vi "Subpanel UI.vi"(8 "error in (no error)":errorcluster, 10 "Message Queue":refnum<queue>, 11 "Pump Controller in":refnum<class "Pump Controller.lvclass">) -> (0 "error out":errorcluster, 3 "Pump Controller out":refnum<class "Pump Controller.lvclass">)   [LabVIEW 2020, in "Pump Controller.lvclass"]
doc: "The UI that will be inserted into subpanels so data can be displayed to the user. The class will use an internally managed message queue to communicate to it. The user should only communicate to this UI through class methods."
uses:
  Pump Controller.lvclass
  Pump Controller.lvclass/Pump Controller.ctl
  Sub VIs/Message Queue/test Message Queue.lvlib
  Sub VIs/Message Queue/Enqueue Message (Single).vi
  <vilib>/Utility/error.llb/Error Cluster From Error Code.vi
  <vilib>/ErrorRing/Error Ring.xnode
  Sub VIs/Message Queue/Message Cluster.ctl
panel:
  out "Name":string
  out "Fault":bool
  out "Running?":bool
  out "Pressure (psi)":dbl format="%#.0f"
  out "Flow Rate (mL/min)":dbl format="%.3f"
  in  "Time Interval (sec)":i32=1200
  out "Pressure Graph":cluster{timestamp[], dbl[]}[](graph)
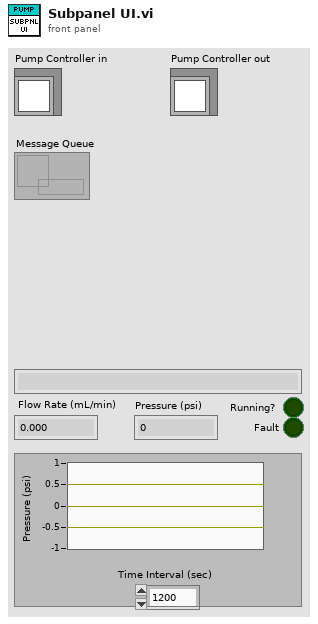
[diagram p1: front panel]
types:
  T1 = cluster{"Data Timestamps":timestamp[], "Data Values":dbl[], "Previous Run State":bool}
  T2 = typedef "Pump Controller.lvclass/Pump Controller State.ctl" = cluster{"VISA Resource":refnum<visa-resource-name>, "Flow Rate":dbl, "Running":bool, "Running Since":timestamp, "Pressure Data Point":cluster{"Time Stamp":timestamp, "Value":dbl}, "Fault":bool, "Sampling Rate (sec/sample)":dbl}
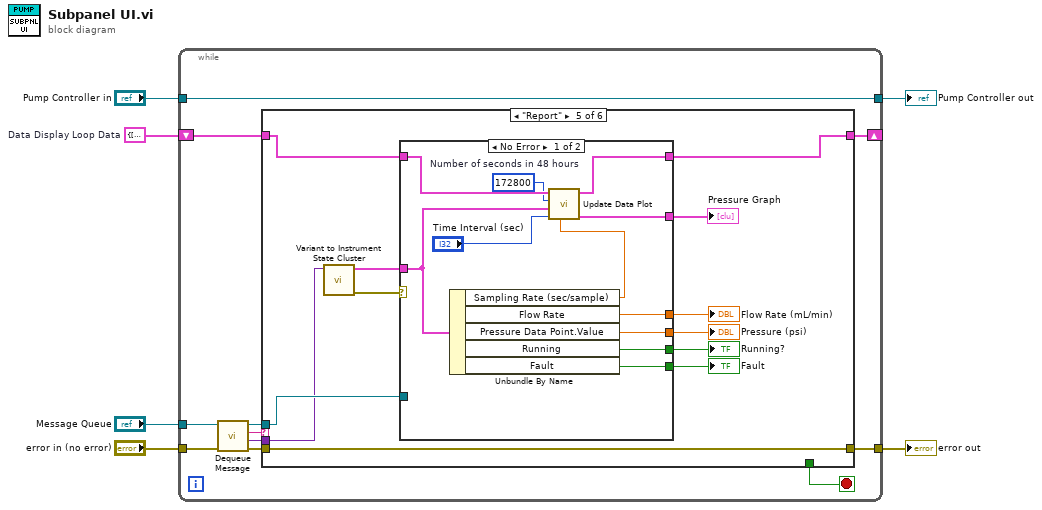
[diagram p0: block diagram]
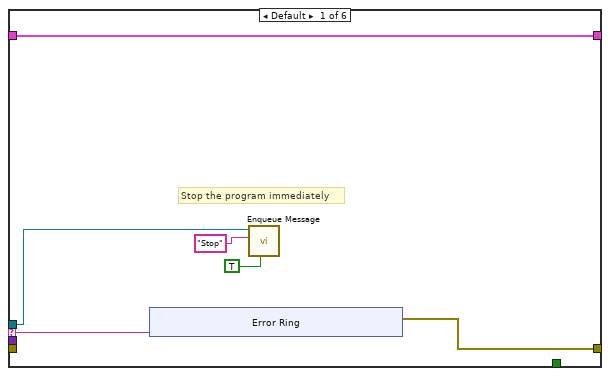
[diagram p2: hidden frame]
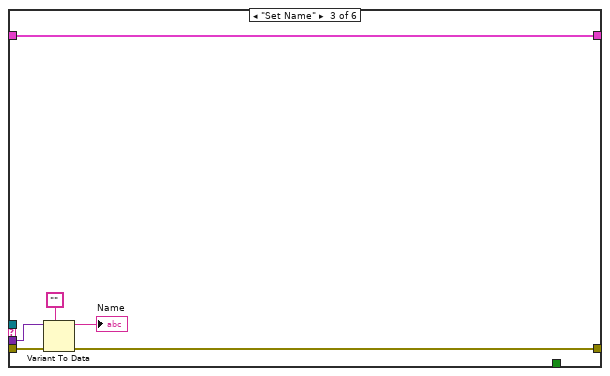
[diagram p4: hidden frame]
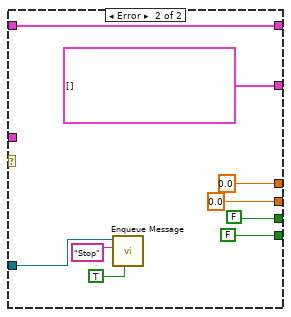
[diagram p6: hidden frame]
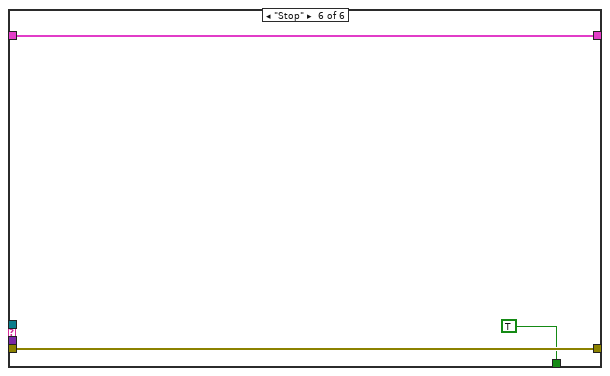
[diagram p7: hidden frame]
diagram:
  w1 = T1 {"Data Timestamps"=[], "Data Values"=[], "Previous Run State"=FALSE}  # Data Display Loop Data
  n1 = while {
    tunnel: [w7] -> w5
    tunnel: "Pump Controller in" -> [w7]
    tunnel: [w11] -> w3
    tunnel: "error in (no error)" -> [w17]
    tunnel: "Message Queue" -> [w16]
    shift-right: [w8] -> _
    shift-left: w1 -> [w9]
    stop <- w10 stop-if-true
    n2 = call "Dequeue Message.vi"("error in (no error)"=w17, "Message Queue"=w16) -> ("error out"=w12:errorcluster, "Message Data"=w14:variant, "Message"=w15:string, "dup Message Queue"=w13:refnum<queue>)  [unwired: 6 in]
    n3 = case shown="\"Report\"" w15 {
      selector: w15 -> [w19 _ _ _ _ _]
      tunnel: w14 -> [_ _ w35 _ w45 _]
      tunnel: w13 -> [w20 _ _ _ w47 _]
      tunnel: w12 -> [_ w32 w38 w40 w52 w75]
      tunnel: [w18 w32 w36 w40 w52 w75] -> w11
      tunnel: [_ _ _ _ _ TRUE] -> w10
      tunnel: w9 -> [w23 w31 w37 w39 w51 w73]
      tunnel: [w23 w31 w37 w39 w50 w73] -> w8
      frame Default {
        # "Stop the program immediately"
        n4 = xnode "Error Ring"("parameter 0"=w19) -> ("error out"=w18:errorcluster)
        n5 = call-poly "Enqueue Message.vi"("Priority Message? (F)"=TRUE, "Message"="Stop", "Message Queue"=w20) -> ()  [unwired: 7 in, 2 out]
      }
      frame "--- Copy this frame ---" {
      }
      frame "Set Name" {
        n6 = Variant To Data(error in=w38, type="", Variant=w35) -> (data=→"Name":string, error out=w36:errorcluster)
      }
      frame "Initialize" {
      }
      frame "Report" {
        n7 = call "Variant to Instrument State Cluster.vi"("Message Data"=w45) -> ("error out"=w48:errorcluster, "Instrument State"=w49:T2)  [unwired: 9 in]
        n8 = case shown="No Error" w48 {
          tunnel: w51 -> [w56 w72]
          tunnel: [w63 w72] -> w50
          tunnel: [w62 cluster{timestamp[], dbl[]}[] [] ("Updated Plot History")] -> w46
          tunnel: w49 -> [w61 _]
          tunnel: [w60 0.0 ("Setpoint")] -> w41
          tunnel: [w59 0.0 ("Current Temperature")] -> w42
          tunnel: [w58 FALSE ("Running")] -> w43
          tunnel: w47 -> [_ w67]
          tunnel: [w55 FALSE ("Fault")] -> w44
          frame No Error {
            w54 = 172800  # Number of seconds in 48 hours
            n9 = Unbundle By Name(w61) -> ("Sampling Rate (sec/sample)"=w53:dbl, "Flow Rate"=w60:dbl, "Pressure Data Point.Value"=w59:dbl, "Running"=w58:bool, "Fault"=w55:bool)
            n10 = call "Update Data Plot.vi"("Sample Rate (sec/sample)"=w53, "Time interval (s)"="Time Interval (sec)", "Pump Controller State"=w61, "History length (-1; unlimited)"=w54, "Graph History Arrays in"=w56) -> ("Updated Plot History"=w62:cluster{timestamp[], dbl[]}[], "Graph History Arrays out"=w63:T1)  [unwired: 5 in]
          }
          frame Error {
            n11 = call-poly "Enqueue Message.vi"("Priority Message? (F)"=TRUE, "Message"="Stop", "Message Queue"=w67) -> ()  [unwired: 7 in, 2 out]
          }
        }
        "Pressure Graph" <- w46
        "Fault" <- w44
        "Running?" <- w43
        "Pressure (psi)" <- w42
        "Flow Rate (mL/min)" <- w41
      }
      frame "Stop" {
      }
    }
  }
  "error out" <- w3
  "Pump Controller out" <- w5
